vi "Coordenadas.vi"() -> ()   [LabVIEW 2016]
panel:
  out "Coordenada_Y":i16[][](array[numeric])
  out "Coordenada_X":i16[][](array[numeric])
  in  "Angulo":i32 min=0 max=360 step=1
  out "size(s) 2":i32[](array[numeric])
  out "size(s)":i32[](array[numeric])
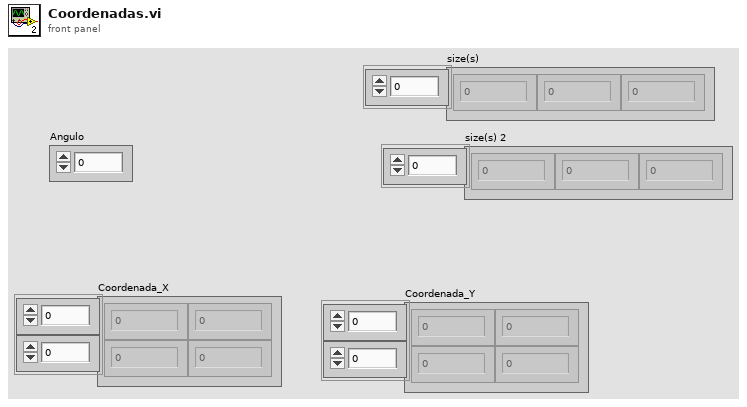
[diagram p1: front panel]
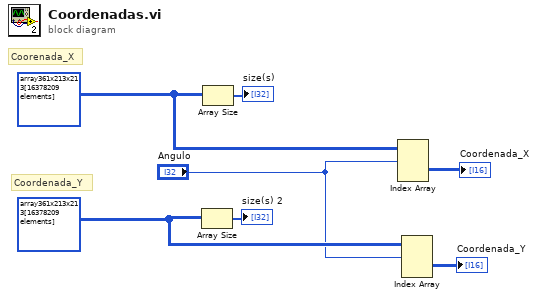
[diagram p0: block diagram]
diagram:
  w4 = i16[][][] array361x213x213[16378209 elements] ("Coordenada_y")
  w5 = i16[][][] array361x213x213[16378209 elements] ("Coordenada_x")
  # "Coorenada_X"
  # "Coordenada_Y"
  n1 = Array Size(array=w4) -> (size(s)=→"size(s) 2":i32[])
  n2 = Array Size(array=w5) -> (size(s)=→"size(s)":i32[])
  n3 = Index Array(array=w5, index (dim 0)="Angulo") -> (element=→"Coordenada_X":i16[][])  [unwired: 2 in]
  n4 = Index Array(array=w4, index (dim 0)="Angulo") -> (element=→"Coordenada_Y":i16[][])  [unwired: 2 in]
